vi "split_str_array.vi"(9 "First  Array":string[](array[string]), 10 "Total Array":string[](array[string])) -> (1 "Rest Array":string[](array[string]))   [LabVIEW 2018]
doc: "Deletes elements in Total Array which belong to First Array, and returns the Rest Array after deletion."
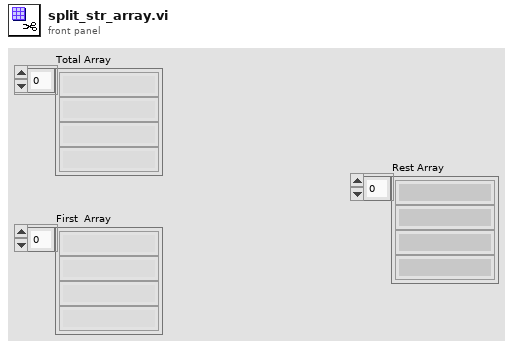
[diagram p1: front panel]
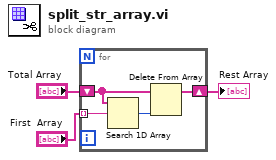
[diagram p0: block diagram]
diagram:
  n1 = for {
    tunnel: "First  Array" -> [w7] mode=indexing
    shift-right: [w5] -> w1
    shift-left: "Total Array" -> [w4]
    n2 = Search 1D Array(1D array=w4, element=w7) -> (index of element=w6:i32)  [unwired: 1 in]
    n3 = Delete From Array(array=w4, index=w6) -> (array with subset deleted=w5:string[])  [unwired: 1 in, 1 out]
  }
  "Rest Array" <- w1
